vi "DC2100 Set LED OnOff.vi"(8 "error in (no error)":errorcluster {"code" format="%.0x"}, 9 "LED On/Off (Off)":bool, 11 "instrument handle":refnum<visa-resource-name>) -> (0 "error out":errorcluster {"code" format="%.0x"}, 3 "instrument handle out":refnum<visa-resource-name>)   [LabVIEW 2019]
doc: "Sets the LED on or off."
uses:
  DC2100_Drv_32.dll
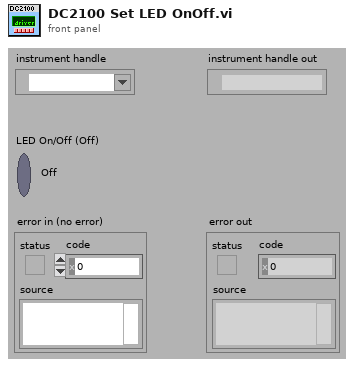
[diagram p1: front panel]
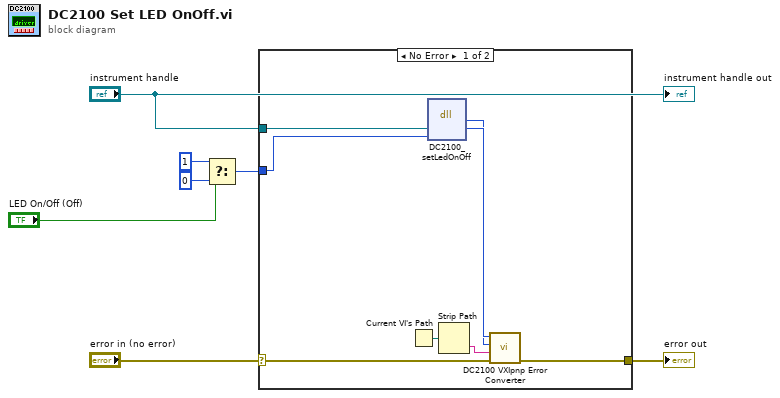
[diagram p0: block diagram]
diagram:
  n1 = Select(t=i16 1, s="LED On/Off (Off)", f=i16 0) -> (s? t:f=w1:i16)
  n2 = case shown="No Error" "error in (no error)" {
    selector: "error in (no error)" -> [w10 w16]
    tunnel: [w9 w16] -> w7
    tunnel: "instrument handle" -> [w14 _]
    tunnel: w1 -> [w8 _]
    frame No Error {
      n3 = Current VI's Path() -> (path=w15:path)
      n4 = dll-call lib="C:/Users/mdrohr/Documents/GitHub/cerebral-hemodynamics/blood-oxygenation/DC2100_Drv_32.dll" fn="DC2100_setLedOnOff"("Instrument Handle"=w14, "LED On/Off"=w8) -> (w12:i32, "Instrument Handle"=w13:u32)  [unwired: 4 in, 2 out]
      n5 = Strip Path(path=w15) -> (name=w11:string)  [unwired: 1 out]
      n6 = call "DC2100 VXIpnp Error Converter.vi"("error in (no error)"=w10, "name of VI (\"\")"=w11, "CVI error code (0)"=w12, "instrument handle"=w13) -> ("error out"=w9:errorcluster)  [unwired: 6 in, 1 out]
    }
    frame Error {
    }
  }
  "error out" <- w7
  "instrument handle out" <- "instrument handle"
